vi "AC Couple (1 Ch SGL Array).vi"(8 "error in (no error)":errorcluster, 10 "Signal":sgl[](array[numeric])) -> (0 "error out":errorcluster, 1 "DC":sgl, 2 "AC Coupled":sgl[](array[numeric]))   [LabVIEW 2017, in "VibrationAnalysisFunctions.lvlib"]
uses:
  <vilib>/addons/InsightCM/Utilities/Analysis/Vibration/VibrationAnalysisFunctions.lvlib
  <vilib>/Analysis/baseanly.llb/Mean (DBL).vi
  <vilib>/Analysis/0measdsp.llb/Scaled Time Domain Window (DBL).vi
  <vilib>/Analysis/NI_AALPro.lvlib
  <vilib>/Analysis/NI_AALBase.lvlib
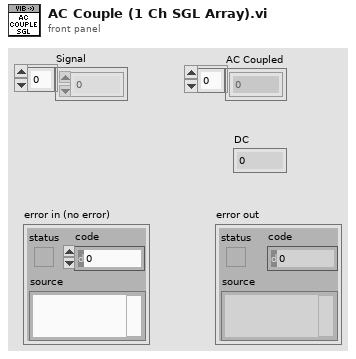
[diagram p1: front panel]
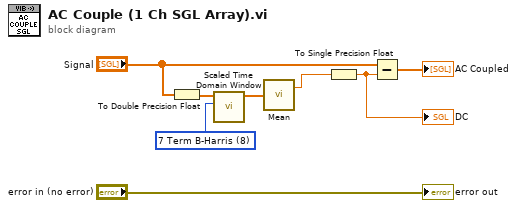
[diagram p0: block diagram]
diagram:
  w7 = u16 8 items=["None ", "Hanning", "Hamming", "Blackman-Harris", "Exact Blackman", "Blackman", "Flat Top", "4 Term B-Harris ", "7 Term B-Harris", "Low Sidelobe"] ("window")
  n1 = To Double Precision Float(number="Signal") -> (double precision float=w5:dbl[])
  n2 = call-poly <vilib>:"Scaled Time Domain Window.vi"("window"=w7, "X"=w5) -> ("Windowed X"=w6:dbl[])  [unwired: 7 in, 2 out]
  n3 = call-poly <vilib>:"Mean.vi"("X"=w6) -> ("mean"=w2:dbl)  [unwired: 1 out]
  n4 = To Single Precision Float(number=w2) -> (single precision float=w1:sgl)
  "DC" <- w1
  n5 = Subtract(x="Signal", y=w1) -> (x-y=→"AC Coupled":sgl[])
  "error out" <- "error in (no error)"
